vi "Translation_Minus.vi"(9 "other Translation":T1, 11 "In Translation":T1) -> (3 "Out Translation":T1)   [LabVIEW 2019, in "Trajectory_Library.lvlib"]
doc: "Subtracts the other translation from the other translation and returns the difference.\n \nFor example, Translation2d{5.0, 4.0} - Translation2d{1.0, 2.0} = Translation2d{4.0, 2.0}\n\nParameters:\n - IN Translation - This translation data structure\n - other Translation - The translation data structure to subtract\n\nReturns\n - Out Translation - The difference between the two translations."
uses:
  Trajectory_Library.lvlib
  TRANSLATION2D.ctl
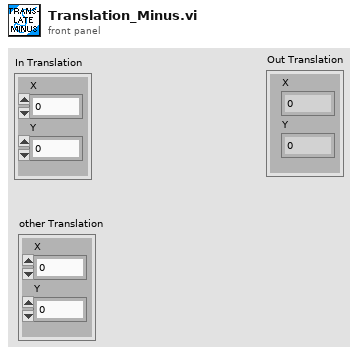
[diagram p1: front panel]
types:
  T1 = typedef "Trajectory_Library.lvlib/TRANSLATION2D.ctl" = cluster{"X":dbl, "Y":dbl}
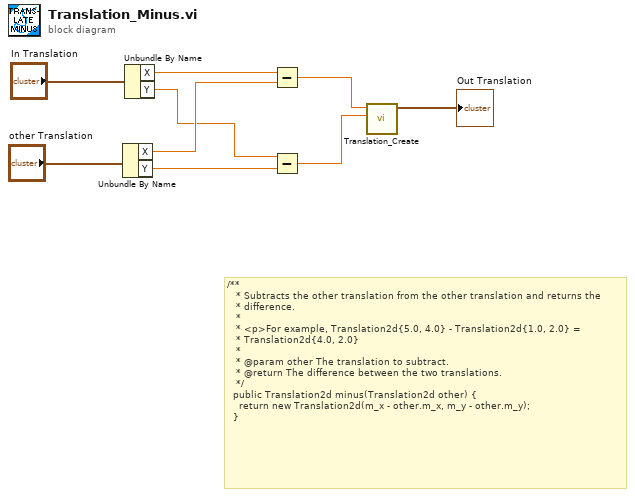
[diagram p0: block diagram]
diagram:
  # "/**\n   * Subtracts the other translation from the other translation and returns the\n   * difference.\n   *\n   * <p>For example, Translation2d{5.0, 4.0} - Translation2d{1.0, 2.0} =\n   * Translation2d{4.0, 2.0}\n   *\n   * @param other The translation to subtract.\n   * @return The difference between the two translations.\n   */\n  public Translation2d minus(Translation2d other) {\n    return new Translation2d(m_x - other.m_x, m_y - other.m_y);\n  }"
  n1 = Unbundle By Name("other Translation") -> ("X"=w6:dbl, "Y"=w5:dbl)
  n2 = Unbundle By Name("In Translation") -> ("X"=w7:dbl, "Y"=w4:dbl)
  n3 = Subtract(x=w7, y=w6) -> (x-y=w2:dbl)
  n4 = Subtract(x=w4, y=w5) -> (x-y=w1:dbl)
  n5 = call "Translation_Create.vi"("Y"=w1, "X"=w2) -> ("TRANSLATION"=→"Out Translation":T1)  [unwired: 9 in]
